vi "GetVIReference.vi"(11 "VI Name To Open":string="Empty.vi") -> (0 "error out":errorcluster, 3 "VI Reference":refnum<vi>)   [LabVIEW 2010]
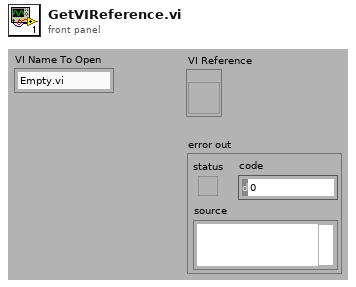
[diagram p1: front panel]
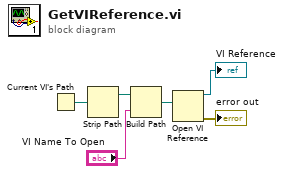
[diagram p0: block diagram]
diagram:
  n1 = Current VI's Path() -> (path=w6:path)
  n2 = Strip Path(path=w6) -> (stripped path=w5:path)  [unwired: 1 out]
  n3 = Build Path(base path=w5, name or relative path="VI Name To Open") -> (appended path=w3:path)
  n4 = Open VI Reference(vi path=w3) -> (vi reference=→"VI Reference":refnum<vi>, error out=→"error out":errorcluster)  [unwired: 5 in]
